vi "Acquire.vi"(7 "Signal Type":T1, 8 "error in":errorcluster, 11 "HW ID in":string) -> (0 "error out":errorcluster, 2 "Graph Data":waveform(dbl)[](array[waveform]), 3 "HW ID out":string)   [LabVIEW 2020, in "Acquisition.lvlib"]
doc: "Perform the acquisition. Replace the contents of this diagram with calls to acquisition hardware.\n_____\nBased on DQMH Project Template 7.0.1.1316."
uses:
  Acquisition.lvlib
  CML Shared/Signal Type--enum.ctl
  CML Shared/CML Shared.lvlib
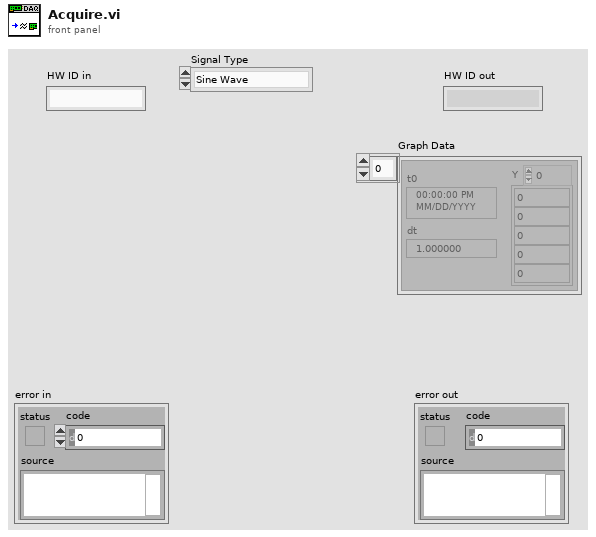
[diagram p1: front panel]
types:
  T1 = typedef "CML Shared.lvlib/Signal Type--enum.ctl" = enum16{"Sine Wave", "Square with Noise"}
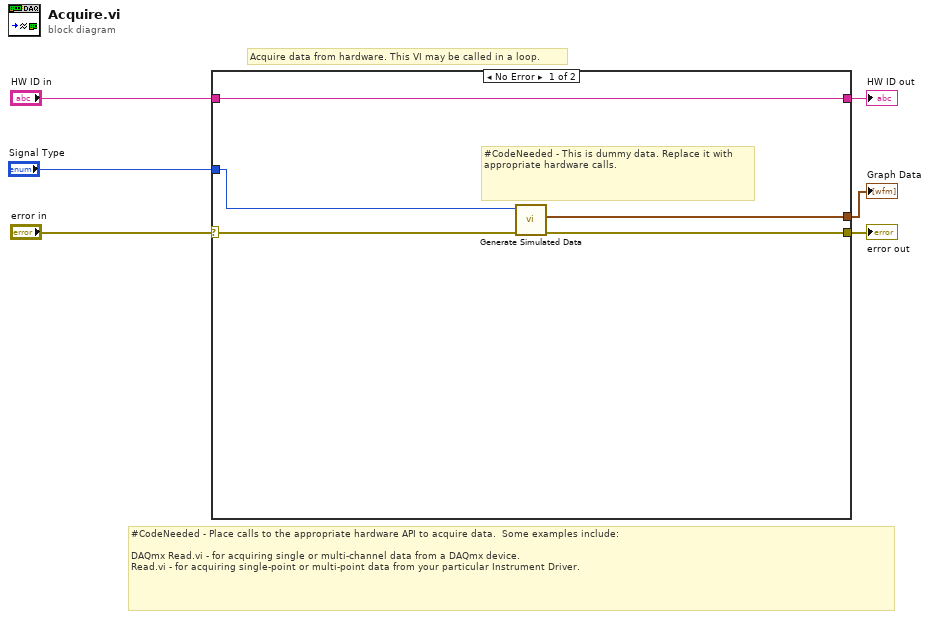
[diagram p0: block diagram]
diagram:
  # "Acquire data from hardware. This VI may be called in a loop."
  # "#CodeNeeded - Place calls to the appropriate hardware API to acquire data.  Some examples include:\n\nDAQmx Read.vi - for acquiring single or multi-channel data from a DAQmx device.\nRead.vi - for acquiring single-point or multi-point data from your particular Instrument Driver."
  n1 = case shown="No Error" "error in" {
    selector: "error in" -> [w11 w12]
    tunnel: [w10 w12] -> w5
    tunnel: "HW ID in" -> [w9 w13]
    tunnel: [w9 w13] -> w3
    tunnel: "Signal Type" -> [w8 _]
    tunnel: [w7 _] -> w1
    frame No Error {
      # "#CodeNeeded - This is dummy data. Replace it with appropriate hardware calls."
      n2 = call "Generate Simulated Data.vi"("error in"=w11, "Signal Type"=w8) -> ("error out"=w10:errorcluster, "Graph Data"=w7:waveform(dbl)[])  [unwired: 8 in]
    }
    frame Error {
    }
  }
  "HW ID out" <- w3
  "error out" <- w5
  "Graph Data" <- w1
